vi "getDevice.vi"(8 "error in (no error)":errorcluster, 10 "Device Number":i32, 11 "Accessory Factory in":refnum<class "Accessory Factory.lvclass">) -> (0 "error out":errorcluster, 1 "AutomatedController":refnum<class "AutomatedController.lvclass">, 3 "Accessory Factory out":refnum<class "Accessory Factory.lvclass">)   [LabVIEW 2020, in "Accessory Factory.lvclass"]
uses:
  Accessory Factory.lvclass
  Devices/AutomatedController/AutomatedController.lvclass
  DeviceFactory/DeviceFactory.lvclass
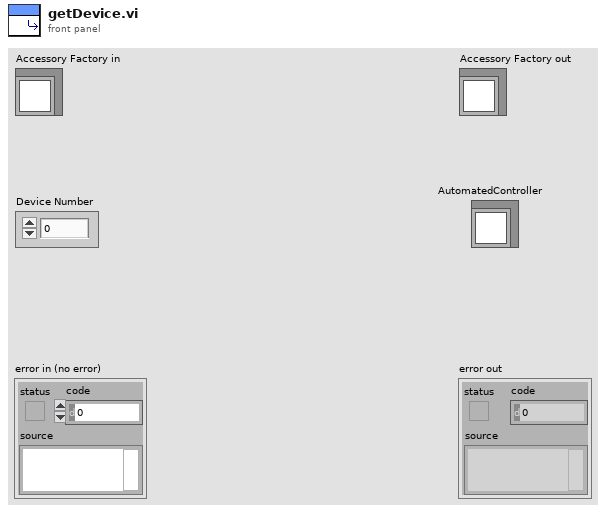
[diagram p1: front panel]
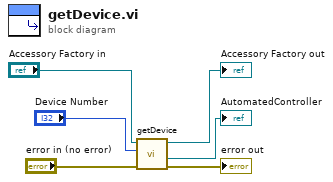
[diagram p0: block diagram]
diagram:
  n1 = call-parent "getDevice.vi"("error in (no error)"="error in (no error)", "Device Number"="Device Number", "DeviceFactory in"="Accessory Factory in") -> ("error out"=→"error out":errorcluster, "AutomatedController"=→"AutomatedController":refnum<class "AutomatedController.lvclass">, "DeviceFactory out"=→"Accessory Factory out":refnum<class "Accessory Factory.lvclass">)  [unwired: 6 in]
